vi "SiggenSafe.vi"(2 "error in (no error)":errorcluster) -> (0 "error out":errorcluster)   [LabVIEW 2009]
doc: "Turn OFF siggen RF."
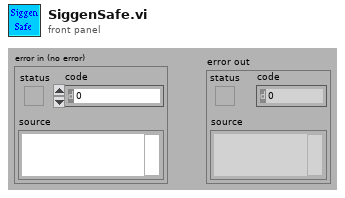
[diagram p1: front panel]
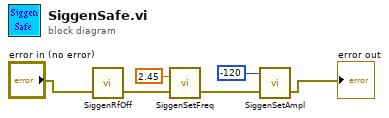
[diagram p0: block diagram]
diagram:
  n1 = call "SiggenRfOff.vi"("error in (no error)"="error in (no error)") -> ("error out"=w2:errorcluster)  [unwired: 2 in]
  n2 = call "SiggenSetFreq.vi"("error in (no error)"=w2, "Freq request (GHz)"=2.45) -> ("Error status"=w4:errorcluster)  [unwired: 1 out]
  n3 = call "SiggenSetAmpl.vi"("error in (no error)"=w4, "Amplitude request (dBm)"=-120) -> ("error out"=→"error out":errorcluster)  [unwired: 1 out]
